vi "Create Analog Replay Listbox IP Text.vi"(8 "error in (no error)":errorcluster, 10 "rios and analog replays":T1(array[cluster]), 11 "Section Ref in":T2 format="%.0x") -> (0 "error out":errorcluster, 2 "listbox text":string[][](array[string]), 3 "Section Ref out":T2 format="%.0x", 5 "not present item indexes":i32[](array[numeric]))   [LabVIEW 2015, in "Engine Simulation Toolkit System Explorer.lvlib"]
uses:
  Engine Simulation Toolkit System Explorer.lvlib
  <vilib>/NI Veristand/Custom Device API/Custom Device Item Ref.ctl
  Shared/Properties.vi
  Shared/Constants and GUIDs.vi
  <vilib>/NI Veristand/Custom Device API/Get Item Property (String).vi
  <vilib>/NI Veristand/Custom Device API/Custom Device API.lvlib
  Shared/Engine Simulation Toolkit Shared.lvlib
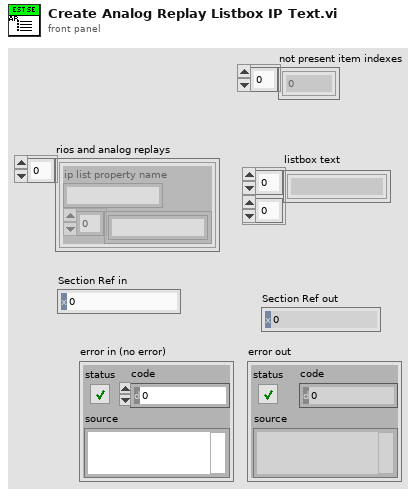
[diagram p1: front panel]
types:
  T1 = cluster{"ip list property name":string, string[]}[]
  T2 = typedef "Custom Device API.lvlib/Custom Device Item Ref.ctl" = u64
  T3 = typedef "Custom Device API.lvlib/Custom Device Item Info.ctl" = cluster{"Name":string, "Is Channel":bool, "GUID":string, "Is Waveform":bool}
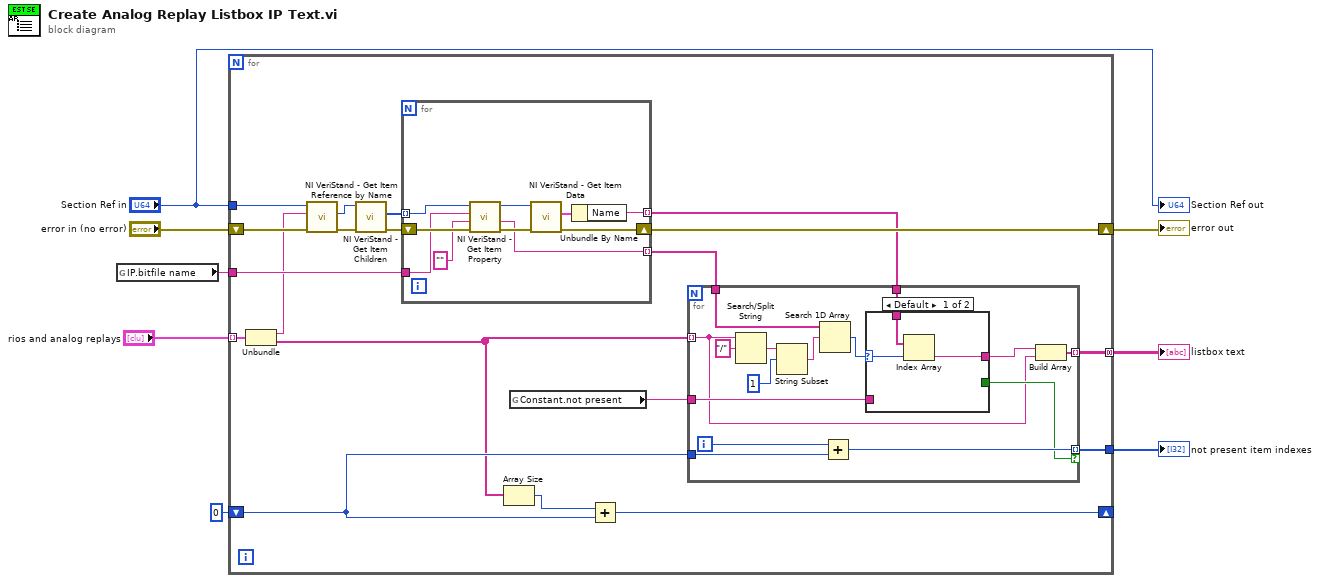
[diagram p0: block diagram]
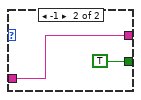
[diagram p2: hidden frame]
diagram:
  n1 = global read "Properties.vi" "IP.bitfile name"() -> (w8:string)
  n2 = for {
    tunnel: w8 -> [w27]
    tunnel: "rios and analog replays" -> [w18] mode=indexing
    tunnel: [w21] -> w7 mode=concatenating
    tunnel: [w24] -> w6
    shift-right: [w26] -> w1
    shift-left: "error in (no error)" -> [w16]
    shift-right: [w20] -> _
    shift-left: 0 -> [w19]
    tunnel: "Section Ref in" -> [w15]
    n3 = Unbundle(w18) -> ("ip list property name"=w14:string, w9:string[])
    n4 = call <vilib>:"NI VeriStand - Get Item Reference by Name.vi"("error in (no error)"=w16, "Item Name"=w14, "Parent Ref in"=w15) -> ("error out"=w17:errorcluster, "Item Ref"=w11:T2)  [unwired: 5 in, 2 out]
    n5 = call <vilib>:"NI VeriStand - Get Item Children.vi"("error in (no error)"=w17, "Item Ref in"=w11) -> ("error out"=w22:errorcluster, "Child Refs"=w23:T2[])  [unwired: 6 in, 2 out]
    n6 = for {
      shift-right: [w52] -> w26
      shift-left: w22 -> [w57]
      tunnel: w23 -> [w55] mode=indexing
      tunnel: w27 -> [w54]
      tunnel: [w49] -> w13 mode=indexing
      tunnel: [w48] -> w12 mode=indexing
      n7 = call-poly <vilib>:"NI VeriStand - Get Item Property.vi"("error in (no error)"=w57, "Default Value"="", "Property Name"=w54, "Item Ref in"=w55) -> ("error out"=w56:errorcluster, "Value"=w49:string, "Item Ref out"=w51:T2)  [unwired: 4 in, 1 out]
      n8 = call <vilib>:"NI VeriStand - Get Item Data.vi"("error in (no error)"=w56, "Item Ref in"=w51) -> ("error out"=w52:errorcluster, "Item Info"=w50:T3)  [unwired: 6 in, 2 out]
      n9 = Unbundle By Name(w50) -> ("Name"=w48:string)
    }
    n10 = Array Size(array=w9) -> (size(s)=w10:i32)
    n11 = global read "Constants and GUIDs.vi" "Constant.not present"() -> (w25:string)
    n12 = Add(x=w10, y=w19) -> (x+y=w20:i32)
    n13 = for {
      tunnel: w9 -> [w29] mode=indexing
      tunnel: w13 -> [w42]
      tunnel: w12 -> [w40]
      tunnel: [w38] -> w21 mode=indexing
      tunnel: w25 -> [w37]
      tunnel: [w34] -> w24 mode=indexing if=w33
      tunnel: w19 -> [w35]
      i -> [w36]
      n14 = Search/Split String(string=w29, search string/char (-)="/") -> (match + rest of string=w31:string)  [unwired: 1 in, 2 out]
      n15 = String Subset(string=w31, offset (0)=1) -> (substring=w28:string)  [unwired: 1 in]
      n16 = Search 1D Array(1D array=w42, element=w28) -> (index of element=w41:i32)  [unwired: 1 in]
      n17 = Add(x=w36, y=w35) -> (x+y=w34:i32)
      n18 = case shown="Default" w41 {
        selector: w41 -> [w44 _]
        tunnel: [w43 w47] -> w39
        tunnel: w40 -> [w45 _]
        tunnel: w37 -> [_ w47]
        tunnel: [_ TRUE] -> w33
        frame Default {
          n19 = Index Array(array=w45, index=w44) -> (element=w43:string)
        }
        frame -1 {
        }
      }
      n20 = Build Array(w39, w29) -> (w38:string[])
    }
  }
  "error out" <- w1
  "listbox text" <- w7
  "not present item indexes" <- w6
  "Section Ref out" <- "Section Ref in"
